vi "Trim_Selection.vi"(0 "Previous_Value":u8, 1 "Trim_Meas":dbl=11.0 format="%#_6p", 2 "Trim_Meas_Array_In":dbl[](array[numeric]), 3 "Trim_Array_In":u8[](array[numeric]), 4 "Trim_1_Set_In":bool, 5 "Error In":errorcluster, 6 "Trim_Config_Settings_Array":T1=[{"Test_Name"="ODFT_Trim", "Target"=1.9, "Reg_Add_0X00"=81, "Data_LSB"=4, "Data_Length"=4, "Settings"=[8, 9, 10, 11, 12, 13, 14, 15, 0, 1, 2, 3, 4, 5, 6, 7], "MSB_Reg_Add_0X00"=0, "Data_MSB"=0}, {"Test_Name"="HV_Trim", "Target"=39.0, "Reg_Add_0X00"=81, "Data_LSB"=0, "Data_Length"=4, "Settings"=[7, 6, 5, 4, 3, 2, 1, 0, 15, 14, 13, 12, 11, 10, 9, 8], "MSB_Reg_Add_0X00"=0, "Data_MSB"=0}, {"Test_Name"="Freq_Trim", "Target"=20.0, "Reg_Add_0X00"=80, "Data_LSB"=0, "Data_Length"=4, "Settings"=[0, 1, 2, 3, 4, 5, 6, 7, 8, 9, 10, 11, 12, 13, 14, 15], "MSB_Reg_Add_0X00"=0, "Data_MSB"=0}] {"MSB_Reg_Add_0X00" format="%.0x"; "Reg_Add_0X00" format="%.0x"}, 8 "Test_Name":string="Freq_Trim") -> (13 "New Value":u8, 14 "Trim_Select_Complete":bool, 15 "Trim_Meas_Array_Out":dbl[](array[numeric]), 16 "Trim_Array_Out":u8[](array[numeric]), 17 "Trim_1_Set_Out":bool, 19 "Error Out":errorcluster)   [LabVIEW 2013]
uses:
  Controls/Trim_Config_Settings_Array.ctl
  Controls/Trim_Config_Settings.ctl
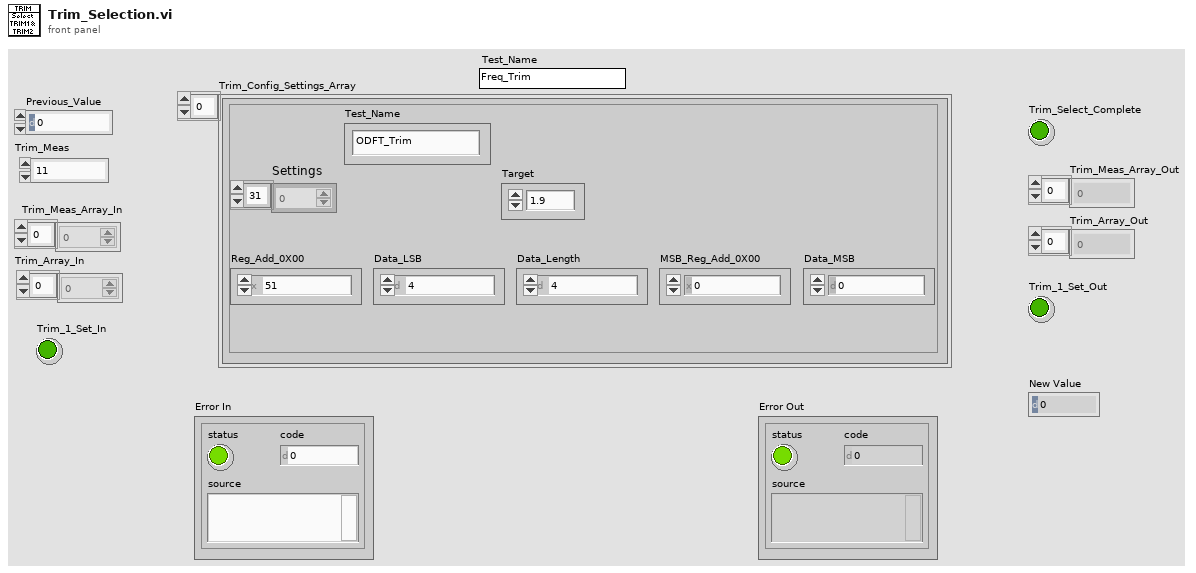
[diagram p1: front panel]
types:
  T1 = typedef "Trim_Config_Settings_Array.ctl" = T2[]
  T2 = typedef "Trim_Config_Settings.ctl" = cluster{"Test_Name":string, "Target":dbl, "Reg_Add_0X00":u8, "Data_LSB":u8, "Data_Length":u8, "Settings":u8[], "MSB_Reg_Add_0X00":u8, "Data_MSB":u8}
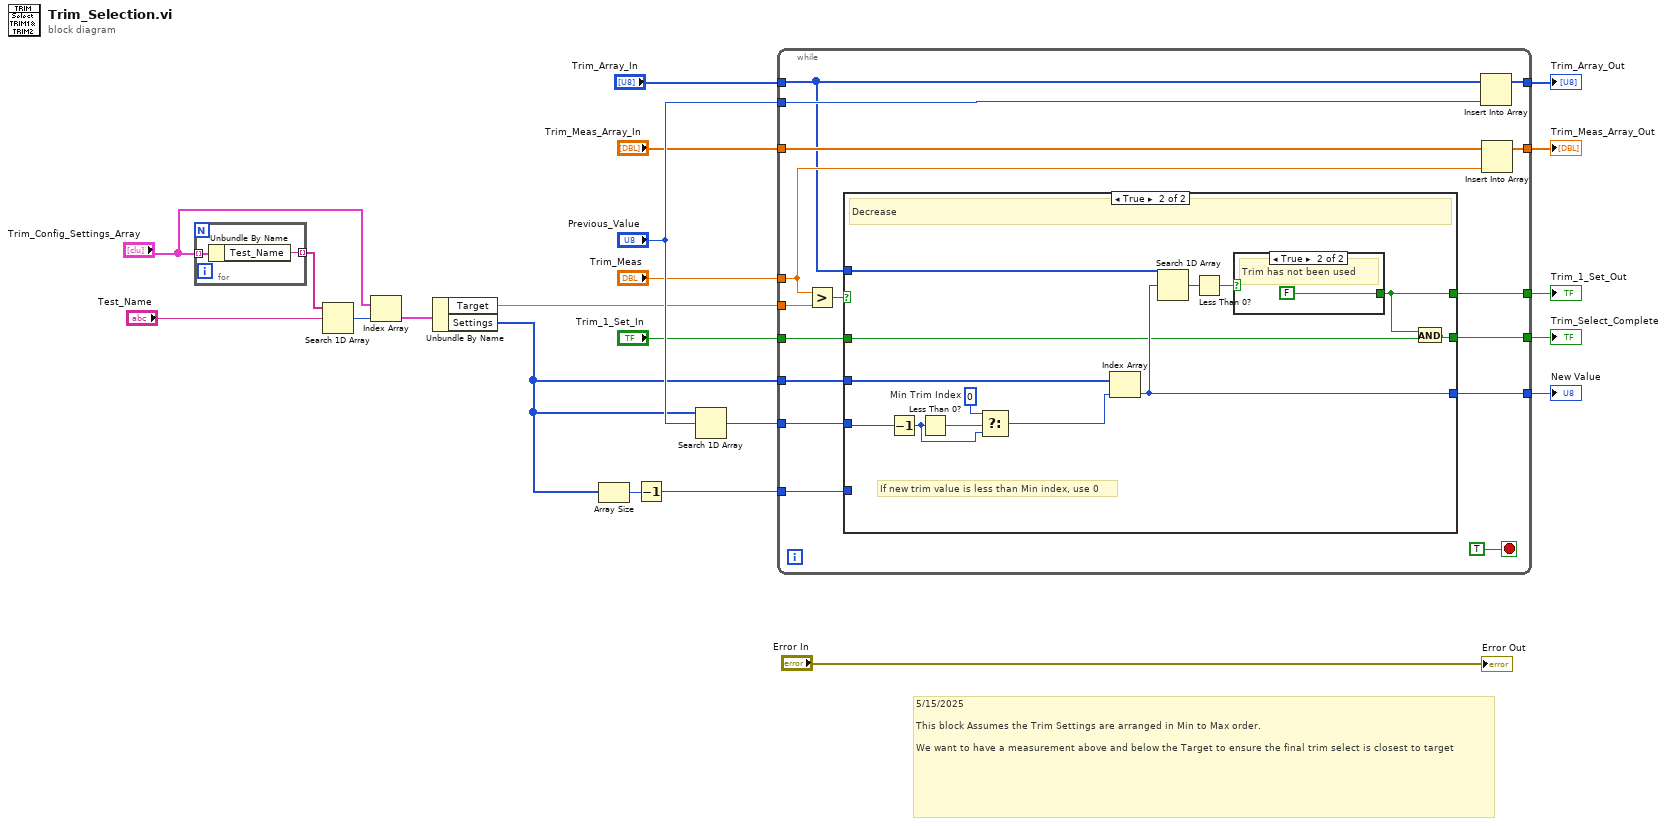
[diagram p0: block diagram]
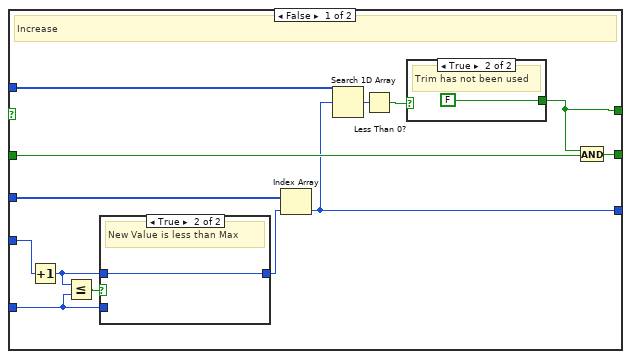
[diagram p2: hidden frame]
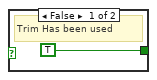
[diagram p4: hidden frame]
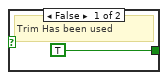
[diagram p5: hidden frame]
diagram:
  # "5/15/2025\n\nThis block Assumes the Trim Settings are arranged in Min to Max order.\n\nWe want to have a measurement above and below the Target to ensure the final trim select is closest to target"
  n1 = for {
    tunnel: "Trim_Config_Settings_Array" -> [w23] mode=indexing
    tunnel: [w22] -> w21 mode=indexing
    n2 = Unbundle By Name(w23) -> ("Test_Name"=w22:string)
  }
  n3 = Search 1D Array(1D array=w21, element="Test_Name") -> (index of element=w19:i32)  [unwired: 1 in]
  n4 = Index Array(array="Trim_Config_Settings_Array", index=w19) -> (element=w18:T2)
  n5 = Unbundle By Name(w18) -> ("Target"=w2:dbl, "Settings"=w11:u8[])
  n6 = Array Size(array=w11) -> (size(s)=w12:i32)
  n7 = Decrement(x=w12) -> (x-1=w7:i32)
  n8 = Search 1D Array(1D array=w11, element="Previous_Value") -> (index of element=w3:i32)  [unwired: 1 in]
  n9 = while {
    tunnel: w11 -> [w32]
    tunnel: "Trim_Meas" -> [w31]
    tunnel: [w38] -> w15
    tunnel: "Trim_Meas_Array_In" -> [w37]
    tunnel: [w36] -> w14
    tunnel: "Trim_Array_In" -> [w28]
    tunnel: w3 -> [w33]
    tunnel: "Previous_Value" -> [w35]
    tunnel: w2 -> [w30]
    tunnel: "Trim_1_Set_In" -> [w29]
    tunnel: w7 -> [w25]
    tunnel: [w27] -> w6
    tunnel: [w26] -> w5
    tunnel: [w24] -> w4
    stop <- TRUE stop-if-true
    n10 = Greater?(x=w31, y=w30) -> (0:w34:bool)
    n11 = case shown="True" w34 {
      tunnel: w33 -> [w41 w58]
      tunnel: w32 -> [w44 w69]
      tunnel: w29 -> [w45 w62]
      tunnel: w28 -> [w47 w68]
      tunnel: [w46 w64] -> w27
      tunnel: [w40 w63] -> w26
      tunnel: w25 -> [w43 _]
      tunnel: [w42 w65] -> w24
      frame False {
        # "Increase"
        n12 = Increment(x=w41) -> (x+1=w49:i32)
        n13 = Less Or Equal?(x=w49, y=w43) -> (x <= y?=w50:bool)
        n14 = case shown="True" w50 {
          tunnel: [w53 w54] -> w48
          tunnel: w49 -> [_ w54]
          tunnel: w43 -> [w53 _]
          frame False {
            # "New Trim Value Exceeds Max"
          }
          frame True {
            # "New Value is less than Max"
          }
        }
        n15 = Index Array(array=w44, index=w48) -> (element=w42:u8)
        n16 = Search 1D Array(1D array=w47, element=w42) -> (index of element=w52:i32)  [unwired: 1 in]
        n17 = Less Than 0?(x=w52) -> (x < 0?=w51:bool)
        n18 = case shown="True" w51 {
          tunnel: [TRUE FALSE] -> w40
          frame False {
            # "Trim Has been used"
          }
          frame True {
            # "Trim has not been used"
          }
        }
        n19 = And(x=w40, y=w45) -> (x .and. y?=w46:bool)
      }
      frame True {
        w60 = u8 0  # Min Trim Index
        # "If new trim value is less than Min index, use 0"
        # "Decrease"
        n20 = Decrement(x=w58) -> (x-1=w61:i32)
        n21 = Less Than 0?(x=w61) -> (x < 0?=w59:bool)
        n22 = Select(t=w60, s=w59, f=w61) -> (s? t:f=w57:i32)
        n23 = Index Array(array=w69, index=w57) -> (element=w65:u8)
        n24 = Search 1D Array(1D array=w68, element=w65) -> (index of element=w67:i32)  [unwired: 1 in]
        n25 = Less Than 0?(x=w67) -> (x < 0?=w66:bool)
        n26 = case shown="True" w66 {
          tunnel: [TRUE FALSE] -> w63
          frame False {
            # "Trim Has been used"
          }
          frame True {
            # "Trim has not been used"
          }
        }
        n27 = And(x=w63, y=w62) -> (x .and. y?=w64:bool)
      }
    }
    n28 = Insert Into Array(array=w28, new element=w35) -> (w36:u8[])  [unwired: 1 in]
    n29 = Insert Into Array(array=w37, new element=w31) -> (w38:dbl[])  [unwired: 1 in]
  }
  "New Value" <- w4
  "Trim_Select_Complete" <- w6
  "Trim_Meas_Array_Out" <- w15
  "Trim_Array_Out" <- w14
  "Trim_1_Set_Out" <- w5
  "Error Out" <- "Error In"
